vi "Z900_navX_Open_I2C.vi"(8 "error in (no error)":errorcluster, 10 "I2C Bus":T1=enum."Invalid", 11 "Update Rate (4Hz - 100Hz)":u8) -> (0 "error out":errorcluster, 3 "navX Library v3.lvlib:navX.lvclass":refnum<class "navX.lvclass">)   [LabVIEW 2015, in "navX Library v3.lvlib" / "navX.lvclass"]
uses:
  navX.lvclass
  <vilib>/Rock Robotics/SystemInterfaces/i2clib/i2c_bus.ctl
  navX Library v2/_TypeDefs/Z900_navX_ProtocolTypeDef.ctl
  navX Library v2/navX Library v2.lvlib
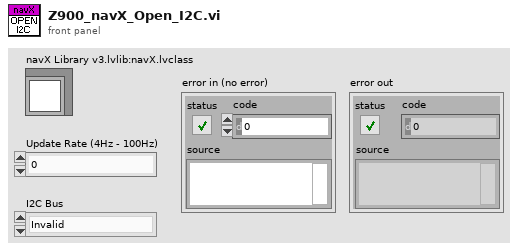
[diagram p1: front panel]
types:
  T1 = typedef "i2c_bus.ctl" = enum16{"I2C On-Board", "I2C MXP", "Invalid"}
  T2 = typedef "navX Library v2.lvlib/Z900_navX_ProtocolTypeDef.ctl" = enum16{"SERIAL", "I2C", "SPI"}
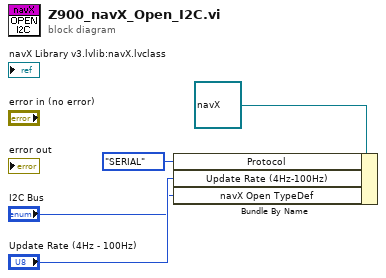
[diagram p0: block diagram]
diagram:
  n1 = Bundle By Name(cluster=refnum<class "navX.lvclass"> refnum ("navX Library v3.lvlib:navX.lvclass"), "Protocol"=Z900_navX_ProtocolTypeDef."SERIAL" ("Interface.Protocol"), "Update Rate (4Hz-100Hz)"="Update Rate (4Hz - 100Hz)", "navX Open TypeDef"="I2C Bus") -> ()  [unwired: 1 out]
